vi "stopDO_img.vi"   [LabVIEW 2015]
uses:
  waveforms/usedDOindepofwf.vi
  Objects/2pparameters.vi
  Objects/configuration.vi
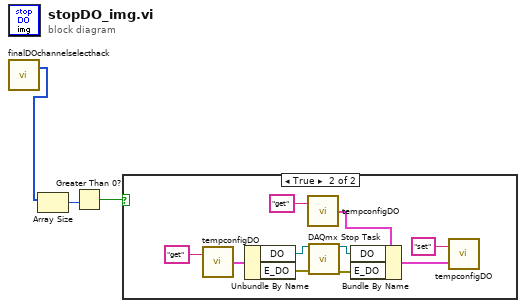
[diagram p0: block diagram]
diagram:
  n1 = call "finalDOchannelselecthack.vi"() -> ("usedDO"=w1:u32[])  [unwired: 1 in, 1 out]
  n2 = Array Size(array=w1) -> (size(s)=w3:i32)
  n3 = Greater Than 0?(x=w3) -> (x > 0?=w2:bool)
  n4 = case shown="True" w2 {
    frame False {
    }
    frame True {
      n5 = call "tempconfigDO.vi"("command"="get") -> ("Temp Config out"=w10:cluster{"DO":refnum<k21>, "E_DO":errorcluster})  [unwired: 1 in]
      n6 = Unbundle By Name(w10) -> ("DO"=w7:refnum<k21>, "E_DO"=w6:errorcluster)
      n7 = call "tempconfigDO.vi"("command"="get") -> ("Temp Config out"=w9:cluster{"DO":refnum<k21>, "E_DO":errorcluster})  [unwired: 1 in]
      n8 = call <vilib>:"DAQmx Stop Task.vi"("task/channels in"=w7, "error in"=w6) -> ("task out"=w5:refnum<k21>, "error out"=w4:errorcluster)  [unwired: 12 in]
      n9 = Bundle By Name(cluster=w9, "DO"=w5, "E_DO"=w4) -> (w8:cluster{"DO":refnum<k21>, "E_DO":errorcluster})
      n10 = call "tempconfigDO.vi"("Temp Config in"=w8, "command"="set") -> ()  [unwired: 1 out]
    }
  }
